vi "change theirs path.vi"(10 "theirs path":string="C:\\Users\\inigo\\Documents\\Kbiosystems\\ColonyPickerProject\\Source_K6-3_Source_JJ-May-22nd-5 40-pm", 11 "Path in":path) -> (3 "path out":path)   [LabVIEW 2022 SP3]
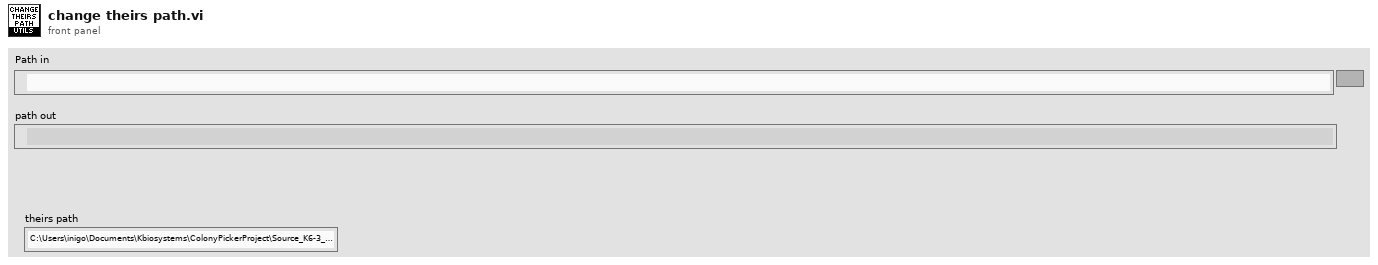
[diagram p1: front panel]
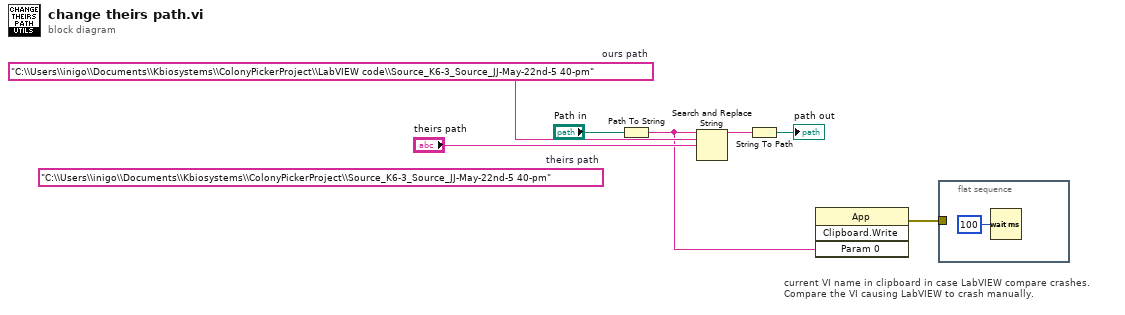
[diagram p0: block diagram]
diagram:
  (unwired) "C:\\Users\\inigo\\Documents\\Kbiosystems\\ColonyPickerProject\\Source_K6-3_Source_JJ-May-22nd-5 40-pm"  # theirs path
  w6 = "C:\\Users\\inigo\\Documents\\Kbiosystems\\ColonyPickerProject\\LabVIEW code\\Source_K6-3_Source_JJ-May-22nd-5 40-pm"  # ours path
  # "current VI name in clipboard in case LabVIEW compare crashes.\nCompare the VI causing LabVIEW to crash manually."
  n1 = Path To String(path="Path in") -> (string=w2:string)
  n2 = Search and Replace String(input string=w2, search string=w6, replace string="theirs path") -> (result string=w3:string)  [unwired: 5 in, 3 out]
  n3 = String To Path(string=w3) -> (path=→"path out":path)
  n4 = invoke class="App" method="Clipboard.Write"("Param 0"=w2) -> (error out=w1:errorcluster)  [unwired: 3 in, 3 out]
  n5 = flat-sequence {
    tunnel: w1 -> [_]
    frame #0 {
      n6 = Wait (ms)(milliseconds to wait=u32 100) -> ()  [unwired: 1 out]
    }
  }
